vi "Configure Autozero.vi"(7 "Auto Zero (0: Enable)":u32(ring) items=["Enable", "Disable", "Once"], 8 "error in (no error)":errorcluster, 9 "Channel List(\"\")":string, 10 "Function (0: Voltage DC)":i32(ring) items=[" Voltage DC"=0, "Current DC"=2, "Resistance"=4, "4-wire Resistance"=5, "Diode"=6, "Temperature"=8, "Voltage Ratio"=12], 11 "VISA resource name":refnum<visa-resource-name>) -> (0 "error out":errorcluster, 3 "VISA resource name out":refnum<visa-resource-name>)   [LabVIEW 2023, in "Keithley DMM6500 DAQ6500 Series.lvlib"]
doc: "Enables or disables the autozero function on the instrument. Enabling autozero optimizes the instrument for accuracy, while disabling optimizes for speed."
uses:
  <instrlib>/Keithley DMM6500 DAQ6500 Series/Keithley DMM6500 DAQ6500 Series.lvlib
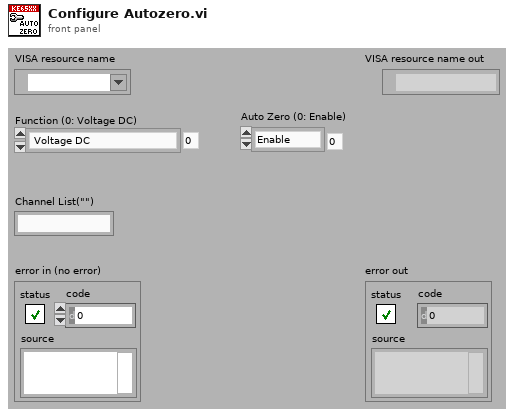
[diagram p1: front panel]
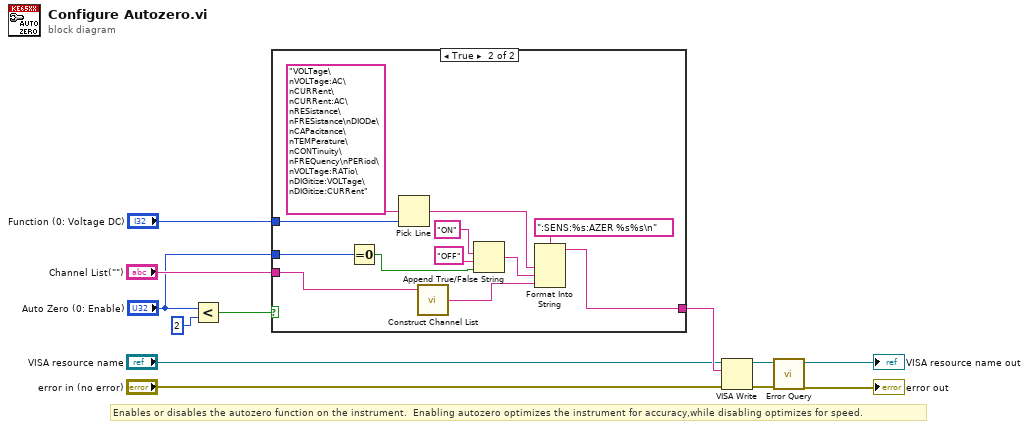
[diagram p0: block diagram]
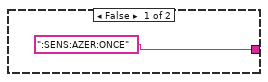
[diagram p2: hidden frame]
diagram:
  # "Enables or disables the autozero function on the instrument.  Enabling autozero optimizes the instrument for accuracy,while disabling optimizes for speed."
  n1 = Less?(x="Auto Zero (0: Enable)", y=u32 2) -> (x < y?=w2:bool)
  n2 = case shown="True" w2 {
    tunnel: [":SENS:AZER:ONCE" w21] -> w12
    tunnel: "Function (0: Voltage DC)" -> [_ w19]
    tunnel: "Channel List(\"\")" -> [_ w17]
    tunnel: "Auto Zero (0: Enable)" -> [_ w15]
    frame False {
    }
    frame True {
      n3 = Equal To 0?(x=w15) -> (x = 0?=w14:bool)
      n4 = Pick Line(multi-line string="VOLTage\nVOLTage:AC\nCURRent\nCURRent:AC\nRESistance\nFRESistance\nDIODe\nCAPacitance\nTEMPerature\nCONTinuity\nFREQuency\nPERiod\nVOLTage:RATio\nDIGitize:VOLTage\nDIGitize:CURRent", line index=w19) -> (output string=w18:string)  [unwired: 1 in]
      n5 = call <instrlib>:"Construct Channel List.vi"("Channel List"=w17) -> ("Channel List String"=w16:string)  [unwired: 2 in]
      n6 = Append True/False String(1:w14, 2:"OFF", 3:"ON") -> (0:w22:string)  [unwired: 1 in]
      n7 = Format Into String(format string=":SENS:%s:AZER %s%s\n", w18, w22, w16) -> (resulting string=w21:string)  [unwired: 2 in, 1 out]
    }
  }
  n8 = VISA Write(VISA resource name="VISA resource name", write buffer=w12, error in (no error)="error in (no error)") -> (VISA resource name out=w9:refnum<visa-resource-name>, error out=w8:errorcluster)  [unwired: 1 out]
  n9 = call <instrlib>:"Error Query.vi"("error in (no error)"=w8, "VISA resource name"=w9) -> ("error out"=→"error out":errorcluster, "VISA resource name out"=→"VISA resource name out":refnum<visa-resource-name>)  [unwired: 6 in, 2 out]
